vi "Set Output Values.vi"(6 "Fundamental Frequency (0.0 Hz)":dbl min=0.0 max=1200000.0 format="%^.3e", 7 "Output Value(s) (0 - Amplitude)":u32(ring) items=["Amplitude", "Volts dc or update volts ac", "Volts ac dBm update", "Volts ac or volts dc with 0 Hz", "Volts ac in dBm", "Current dc or update current ac", "Current ac", "Update frequency", "Resistance", "Capacitance", "Temperature (Celsius)", "Temperature (Fahrenheit)", "Power dc or update power ac", "Power ac", "Dual volts dc or update dual ac", "Dual volts ac in volts", "Power ac in dBm update", "Power ac in dBm", "Dual volts ac in dBm update", "Dual volts ac in dBm"], 8 "error in (no error)":errorcluster, 9 "Secondary Value (0.0)":dbl format="%^.3e", 10 "Primary Value (0.0)":dbl format="%^.3e", 11 "VISA resource name":refnum<visa-resource-name>) -> (0 "error out":errorcluster {"code" format="%.0x"}, 3 "VISA resource name out":refnum<visa-resource-name>)   [LabVIEW 2012, in "Fluke 5XXX Series Multicalibrators.lvlib"]
doc: "This VI sets the output of the Calibrator and establishes a new reference point for the error mode. If only one amplitude is supplied, the Calibrator sources a single output. If two amplitudes are supplied, the Calibrator sources two outputs. The second amplitude will be sourced at the AUX terminals for dual voltage outputs. If the frequency is not supplied, the Calibrator will use the frequency that is presently in use.\n\nNotes:\n\n(1) Instrument models 5700A, 5720A and 57LFC are not equipped with dual outpus. Only single output operations are available.\n\n(2) To source or measure a temperature, select the desired sensor and sensor parameters first (instrument models 5500A and 5520A only).\n\n(3) To source a signal using the Calibrator scope options, refer to the Oscilloscope Functions (instrument models 5500A and 5520A only).\n\n(4) If you change the frequency of an ac function and the harmonic output is not explicitly set at the same time with the function Set Harmonic, the harmonic will be set to 1 (instrument models 5500A and 5520A only)."
uses:
  Fluke 5XXX Series Multicalibrators.lvlib
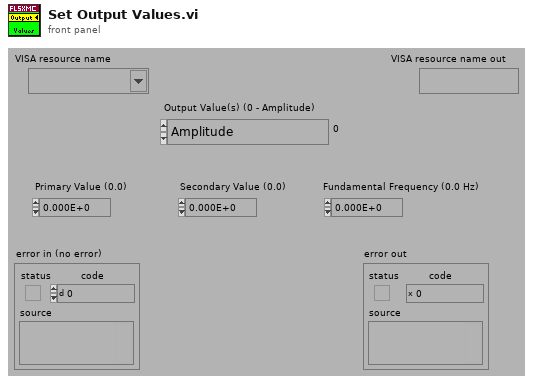
[diagram p1: front panel]
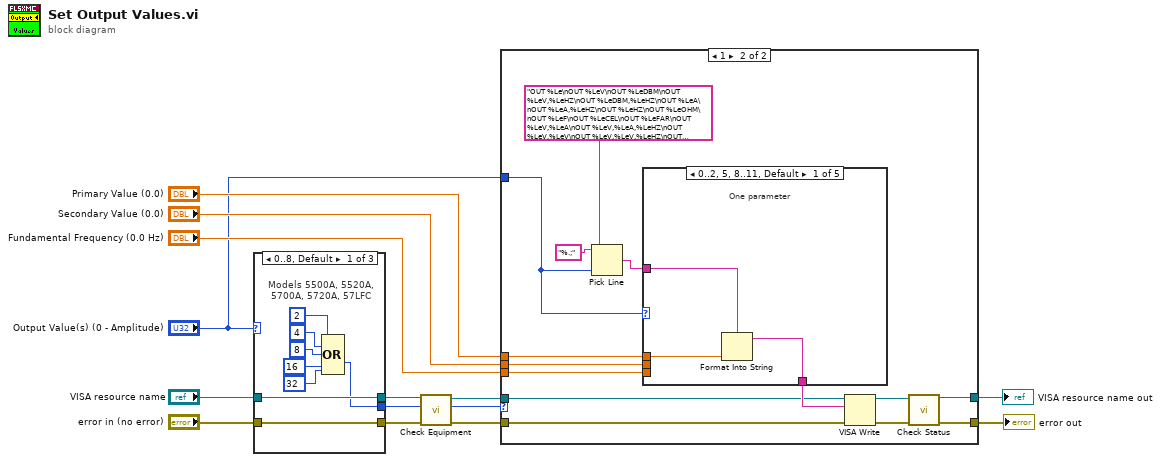
[diagram p0: block diagram]
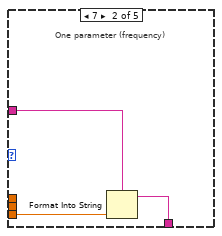
[diagram p3: hidden frame]
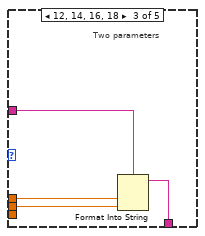
[diagram p4: hidden frame]
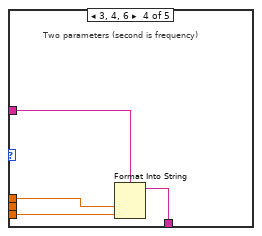
[diagram p5: hidden frame]
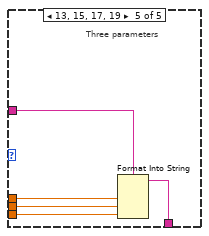
[diagram p6: hidden frame]
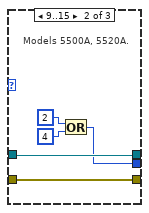
[diagram p7: hidden frame]
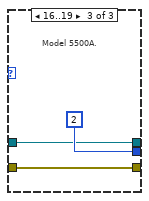
[diagram p8: hidden frame]
diagram:
  n1 = case shown="0..8, Default" "Output Value(s) (0 - Amplitude)" {
    tunnel: "VISA resource name" -> [w17 w25 w29]
    tunnel: "error in (no error)" -> [w18 w23 w28]
    tunnel: [w17 w25 w29] -> w3
    tunnel: [w18 w23 w28] -> w4
    tunnel: [w16 w24 2 ("Numeric")] -> w2
    frame 0..8, Default {
      # "Models 5500A, 5520A,\n 5700A, 5720A, 57LFC"
      n2 = Compound Arithmetic op=OR(u32 2 ("Numeric"), u32 4 ("Numeric"), u32 8 ("Numeric"), u32 16 ("Numeric"), u32 32 ("Numeric")) -> (w16:u32)
    }
    frame 9..15 {
      # "Models 5500A, 5520A."
      n3 = Or(x=2 ("Numeric"), y=4 ("Numeric")) -> (x .or. y?=w24:i32)
    }
    frame 16..19 {
      # "Model 5500A."
    }
  }
  n4 = call "Check Equipment.vi"("error in (no error)"=w4, "Bit Mask"=w2, "VISA resource name"=w3) -> ("error out"=w5:errorcluster, "Present?"=w1:u32, "VISA resource name out"=w6:refnum<visa-resource-name>)  [unwired: 6 in]
  n5 = case shown="1" w1 {
    tunnel: w6 -> [w32 w44]
    tunnel: w5 -> [w31 w43]
    tunnel: [w32 w39] -> w12
    tunnel: [w31 w37] -> w11
    tunnel: "Output Value(s) (0 - Amplitude)" -> [_ w35]
    tunnel: "Primary Value (0.0)" -> [_ w46]
    tunnel: "Fundamental Frequency (0.0 Hz)" -> [_ w42]
    tunnel: "Secondary Value (0.0)" -> [_ w41]
    frame 0, Default {
    }
    frame 1 {
      n6 = Pick Line(string ("")="%.;", multi-line string="OUT %Le\nOUT %LeV\nOUT %LeDBM\nOUT %LeV,%LeHZ\nOUT %LeDBM,%LeHZ\nOUT %LeA\nOUT %LeA,%LeHZ\nOUT %LeHZ\nOUT %LeOHM\nOUT %LeF\nOUT %LeCEL\nOUT %LeFAR\nOUT %LeV,%LeA\nOUT %LeV,%LeA,%LeHZ\nOUT %LeV,%LeV\nOUT %LeV,%LeV,%LeHZ\nOUT %LeDBM,%LeA\nOUT %LeDBM,%LeA,%LeHZ\nOUT %LeDBM,%LeDBM\nOUT %LeDBM,%LeDBM,%LeHZ", line index=w35) -> (output string=w34:string)
      n7 = case shown="0..2, 5, 8..11, Default" w35 {
        tunnel: w46 -> [w49 _ w56 w60 w65]
        tunnel: [w48 w52 w54 w58 w62] -> w45
        tunnel: w42 -> [_ w51 _ w59 w63]
        tunnel: w41 -> [_ _ w55 _ w64]
        tunnel: w34 -> [w47 w50 w53 w57 w61]
        frame 0..2, 5, 8..11, Default {
          # "One parameter"
          n8 = Format Into String(format string=w47, w49) -> (resulting string=w48:string)  [unwired: 2 in, 1 out]
        }
        frame 7 {
          # "One parameter (frequency)"
          n9 = Format Into String(format string=w50, w51) -> (resulting string=w52:string)  [unwired: 2 in, 1 out]
        }
        frame 12, 14, 16, 18 {
          # "Two parameters"
          n10 = Format Into String(format string=w53, w56, w55) -> (resulting string=w54:string)  [unwired: 2 in, 1 out]
        }
        frame 3, 4, 6 {
          # "Two parameters (second is frequency)"
          n11 = Format Into String(format string=w57, w60, w59) -> (resulting string=w58:string)  [unwired: 2 in, 1 out]
        }
        frame 13, 15, 17, 19 {
          # "Three parameters"
          n12 = Format Into String(format string=w61, w65, w64, w63) -> (resulting string=w62:string)  [unwired: 2 in, 1 out]
        }
      }
      n13 = VISA Write(VISA resource name=w44, write buffer=w45, error in (no error)=w43) -> (VISA resource name out=w40:refnum<visa-resource-name>, error out=w38:errorcluster)  [unwired: 1 out]
      n14 = call "Check Status.vi"("VISA resource name"=w40, "error in (no error)"=w38) -> ("VISA resource name out"=w39:refnum<visa-resource-name>, "error out"=w37:errorcluster)  [unwired: 12 in]
    }
  }
  "VISA resource name out" <- w12
  "error out" <- w11
